vi "Read Look Up Table.vi"(11 "Executioner in":refnum<class "Executioner.lvclass">) -> (1 "Attributes Ref":refnum<data-value>, 3 "Executioner out":refnum<class "Executioner.lvclass">)   [LabVIEW 2017, in "Test Executive.lvlib" / "Executioner.lvclass"]
uses:
  <vilib>/gpm_packages/@cs/test-executive/Source/Test Executive/Executioner/Executioner.lvclass
  <vilib>/gpm_packages/@cs/lookup-table/Source/LookupTable/LookupTable.lvclass
  <vilib>/gpm_packages/@cs/test-executive/Source/Test Executive/Executioner/Executioner.lvclass/Executioner.ctl
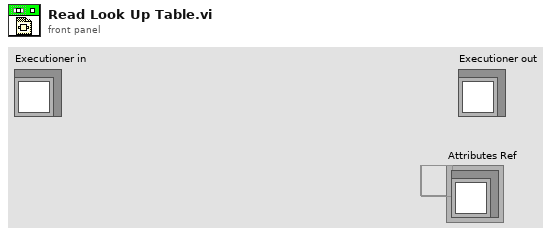
[diagram p1: front panel]
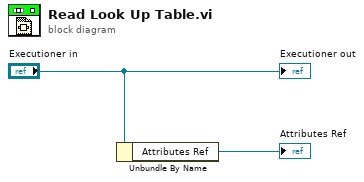
[diagram p0: block diagram]
diagram:
  n1 = Unbundle By Name("Executioner in") -> ("Attributes Ref"=→"Attributes Ref":refnum<data-value>)
  "Executioner out" <- "Executioner in"
